vi "Sensor de Flujo_HEGO_2.vi"() -> ()   [LabVIEW 2015]
uses:
  <vilib>/MakerHub/LINX/Public/Peripherals/Digital/Digital Read N Chans.vi
  <vilib>/MakerHub/LINX/Private/Local IO/LinxDigitalRead.vi
  <vilib>/MakerHub/LINX/Public/Utilities/Check Channel.vi
  <vilib>/MakerHub/LINX/Public/Utilities/Open Serial.vi
  <vilib>/MakerHub/LINX/Private/Utilties/Generate Error.vi
  <vilib>/ptbypt/NI_PtbyPt.lvlib
  <vilib>/MakerHub/LINX/LMH-LINX.lvlib
panel:
  out "x+y":dbl
  in  "Guardar datos a excel":bool
  out "Flujo de Salida":dbl
  in  "Rango de Grafica (tiempo)":u32(knob) scale=0.0..100.0
  in  "tiempo de muestreo":dbl(knob)=0.2 caption="Time Target (s)" scale=0.0..1.0
  out "Numeric 2":i32
  out "NumdePulsos2":i32
  out "XY Graph":cluster{dbl[], dbl[]}[](graph) caption="Flujo de Entrada y Salida"
  out "Loop Rate (Hz)":u32
  in  "Pin del Sensor 2":u8
  in  "Pin del Sensor 1":u8
  in  "Puerto Serial":refnum<visa-resource-name>
  in  "?":bool
  out "Flujo de Entrada":dbl
  out "Numero de puls":i32
  out "NumdePulsos1":i32
  # "MONITOREO DE FLUJO ATRAVEZ DEL SENSOR YF-S201"
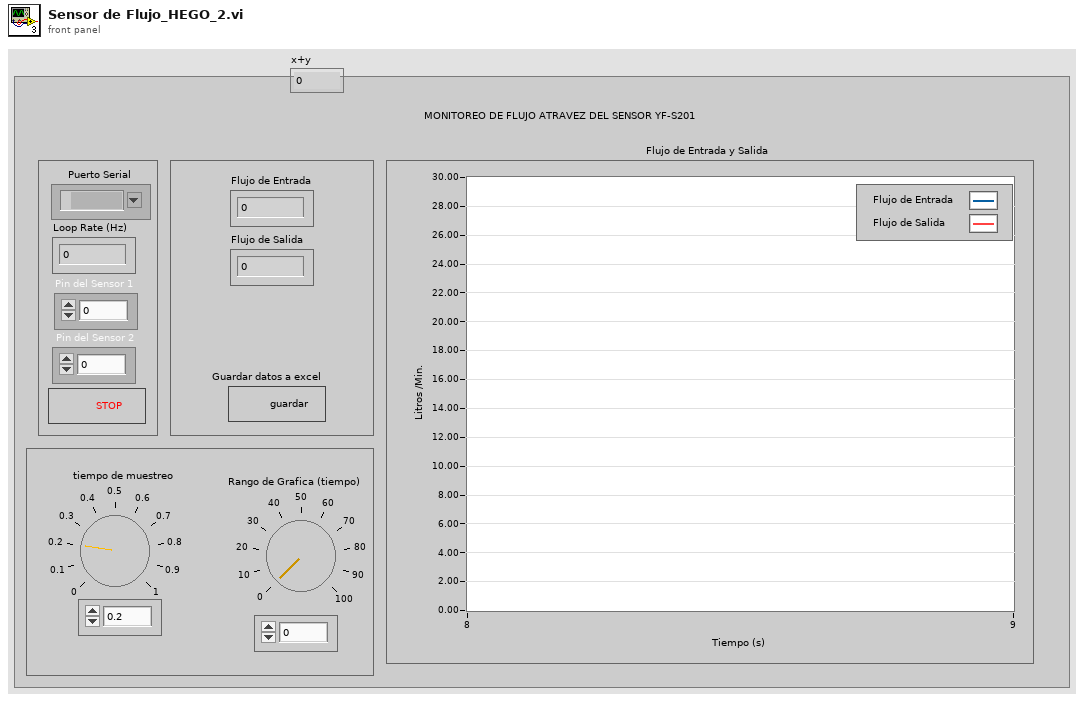
[diagram p1: front panel]
types:
  T1 = typedef "LMH-LINX.lvlib/LINX Ref.ctl" = cluster{"IO":T2, "Interface":T3, "LINX Device Config":T4}
  T2 = typedef "LMH-LINX.lvlib/Platform.ctl" = enum16{"Remote", "Local"}
  T3 = typedef "LMH-LINX.lvlib/Interface.ctl" = enum16{"Serial", "TCP"}
  T4 = typedef "LMH-LINX.lvlib/Device.lvlib/LINX Device Config.ctl" = cluster{"Interface":T3, "COM Port":refnum<visa-resource-name>, "TCP Configuration":T5, "Device Family":u8, "Device ID":u8, "Device Name":string, "TCP Ref":refnum<k5>, "Channels":T6}
  T5 = typedef "LMH-LINX.lvlib/Device.lvlib/TCP Config.ctl" = cluster{"IP Address":string, "Port":u16}
  T6 = typedef "LMH-LINX.lvlib/Channels.ctl" = cluster{"DI":u8[], "DO":u8[], "AI":u8[], "AO":u8[], "PWM":u8[], "QE":u8[], "UART":u8[], "I2C 2":u8[], "SPI":u8[], "CAN":u8[], "Servo":u8[], "AI Ref (V)":dbl, "AI Resolution (Bits)":u8, "AO Ref (V)":dbl, "AO Resolution (Bits)":u8}
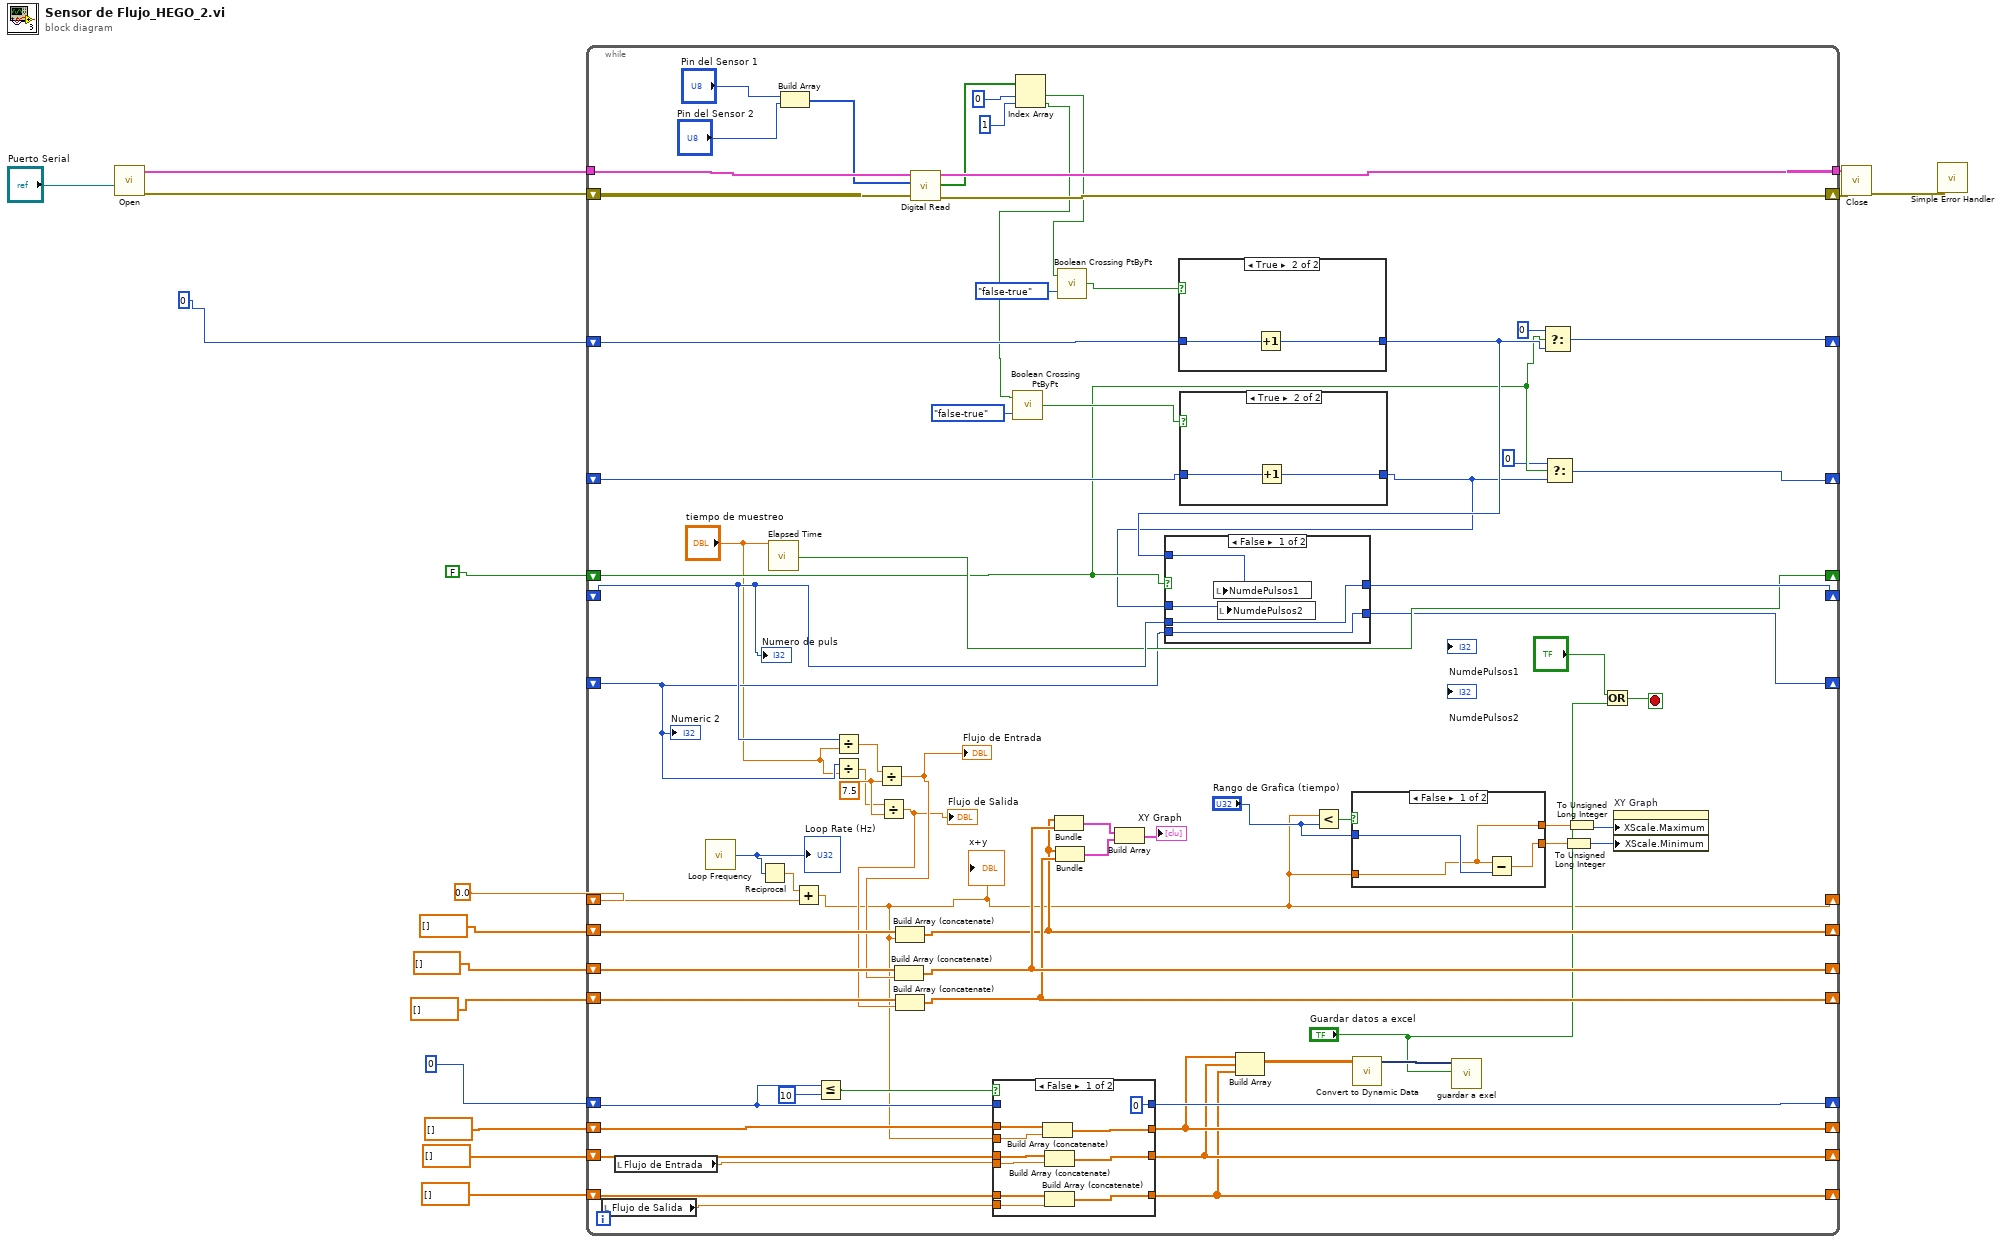
[diagram p0: block diagram]
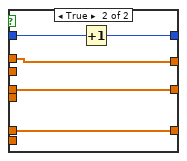
[diagram p2: hidden frame]
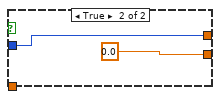
[diagram p3: hidden frame]
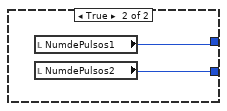
[diagram p5: hidden frame]
diagram:
  n1 = call-poly <vilib>:"Open.vi"("Serial Port"="Puerto Serial") -> ("Error Out"=w15:errorcluster, "LINX Resource"=w16:T1)  [unwired: 8 in, 1 out]
  n2 = while {
    tunnel: w16 -> [w80]
    tunnel: [w81] -> w13
    shift-right: [w83] -> _
    shift-left: 0 ("CONTADOR 2") -> [w86]
    shift-right: [w82] -> _
    shift-left: _ -> [w69]
    shift-right: [w57] -> _
    shift-left: _ -> [w70]
    shift-right: [w68] -> _
    shift-left: FALSE -> [w59]
    shift-right: [w17] -> _
    shift-left: 0.0 -> [w65]
    shift-right: [w43] -> _
    shift-left: dbl[] [] -> [w64]
    shift-right: [w61] -> _
    shift-left: dbl[] [] -> [w63]
    shift-right: [w60] -> _
    shift-left: _ -> [w54]
    shift-right: [w49] -> _
    shift-left: dbl[] [] ("Numeric") -> [w51]
    shift-right: [w44] -> w5
    shift-left: w15 -> [w79]
    shift-right: [w31] -> _
    shift-left: dbl[] [] ("Numeric") -> [w36]
    shift-right: [w32] -> _
    shift-left: dbl[] [] -> [w38]
    shift-right: [w33] -> _
    shift-left: dbl[] [] -> [w37]
    shift-right: [w34] -> _
    shift-left: 0 -> [w35]
    stop <- w28 stop-if-true
    w53 = 7.5
    n3 = local read "Flujo de Salida"() -> (w29:dbl)
    n4 = local read "Flujo de Entrada"() -> (w30:dbl)
    n5 = call <vilib>:"Loop Frequency.vi"() -> ("Loop Rate (Hz)"=w67:u32)
    "Loop Rate (Hz)" <- w67
    n6 = Reciprocal(x=w67) -> (1/x=w66:dbl)
    n7 = call "Elapsed Time"("Time Target (s)"="tiempo de muestreo") -> ("Time has Elapsed"=w68:bool)  [unwired: 11 in, 7 out]
    n8 = Build Array("Pin del Sensor 1", "Pin del Sensor 2") -> (w75:u8[])
    n9 = Add(x=w66, y=w65) -> (x+y=w17:dbl)
    "x+y" <- w17
    n10 = Less Or Equal?(x=w35, y=u32 10) -> (x <= y?=w23:bool)
    n11 = Divide(x=w69, y="tiempo de muestreo") -> (x/y=w55:dbl)
    n12 = Divide(x=w54, y="tiempo de muestreo") -> (x/y=w52:dbl)
    n13 = Divide(x=w55, y=w53) -> (x/y=w62:dbl)
    "Flujo de Entrada" <- w62
    n14 = Divide(x=w52, y=w53) -> (x/y=w42:dbl)
    "Flujo de Salida" <- w42
    n15 = Build Array (concatenate)(w63, w62) -> (w61:dbl[])
    n16 = Build Array (concatenate)(w64, w17) -> (w43:dbl[])
    n17 = Build Array (concatenate)(w51, w42) -> (w49:dbl[])
    n18 = call-poly <vilib>:"Digital Read.vi"("Error In"=w79, "DI Channels"=w75, "LINX Resource"=w80) -> ("Error Out"=w44:errorcluster, "Values"=w74:bool[], "LINX Resource"=w81:T1)  [unwired: 6 in]
    n19 = case shown="False" w23 {
      tunnel: w35 -> [_ w103]
      tunnel: [u32 0 w102] -> w34
      tunnel: w37 -> [w97 w99]
      tunnel: w30 -> [w95 _]
      tunnel: [w98 w101] -> w32
      tunnel: w38 -> [w96 w101]
      tunnel: w29 -> [w93 _]
      tunnel: w36 -> [w94 w100]
      tunnel: [w92 w100] -> w31
      tunnel: [w91 w99] -> w33
      tunnel: w17 -> [w90 _]
      frame False {
        n20 = Build Array (concatenate)(w97, w90) -> (w91:dbl[])
        n21 = Build Array (concatenate)(w96, w95) -> (w98:dbl[])
        n22 = Build Array (concatenate)(w94, w93) -> (w92:dbl[])
      }
      frame True {
        n23 = Increment(x=w103) -> (x+1=w102:u32)
      }
    }
    n24 = Index Array(array=w74, index #1=0 ("index"), index #2=1 ("index")) -> (element #1=w25:bool, element #2=w24:bool)
    n25 = call <vilib>:"Boolean Crossing PtByPt.vi"("direction"=enum16{"either", "false-true", "true-false"}."false-true", "input"=w24) -> ("crossing"=w71:bool)  [unwired: 1 in]
    n26 = Bundle(w43, w61) -> (w50:cluster{dbl[], dbl[]})  [unwired: 1 in]
    n27 = Bundle(w43, w49) -> (w48:cluster{dbl[], dbl[]})  [unwired: 1 in]
    n28 = call <vilib>:"Boolean Crossing PtByPt.vi"("direction"=enum16{"either", "false-true", "true-false"}."false-true", "input"=w25) -> ("crossing"=w87:bool)  [unwired: 1 in]
    n29 = Build Array(w50, w48) -> (→"XY Graph":cluster{dbl[], dbl[]}[])
    n30 = case shown="True" w87 {
      tunnel: w86 -> [w118 w120]
      tunnel: [w118 w119] -> w84
      frame False {
      }
      frame True {
        n31 = Increment(x=w120) -> (x+1=w119:i32)
      }
    }
    n32 = case shown="True" w71 {
      tunnel: w70 -> [w109 w111]
      tunnel: [w109 w110] -> w56
      frame False {
      }
      frame True {
        n33 = Increment(x=w111) -> (x+1=w110:i32)
      }
    }
    n34 = case shown="False" w59 {
      tunnel: w84 -> [w115 _]
      tunnel: [w114 w117] -> w82
      tunnel: w69 -> [w114 _]
      tunnel: w56 -> [w113 _]
      tunnel: [w112 w116] -> w60
      tunnel: w54 -> [w112 _]
      frame False {
        n35 = local write "NumdePulsos1"(w115) -> ()
        n36 = local write "NumdePulsos2"(w113) -> ()
      }
      frame True {
        n37 = local read "NumdePulsos1"() -> (w117:i32)
        n38 = local read "NumdePulsos2"() -> (w116:i32)
      }
    }
    n39 = Build Array(w33, w32, w31) -> (w39:dbl[][])
    n40 = Less?(x=w17, y="Rango de Grafica (tiempo)") -> (x < y?=w45:bool)
    n41 = case shown="False" w45 {
      tunnel: [w104 w107] -> w21
      tunnel: [w106 0.0] -> w20
      tunnel: w17 -> [w104 _]
      tunnel: "Rango de Grafica (tiempo)" -> [w105 w107]
      frame False {
        n42 = Subtract(x=w104, y=w105) -> (x-y=w106:dbl)
      }
      frame True {
      }
    }
    n43 = call "Convert to Dynamic Data"("2D Array"=w39) -> ("Dynamic Data Type"=w40:dynamicdata)  [unwired: 3 in]
    n44 = call "guardar a exel"("Signals"=w40, "Enable"="Guardar datos a excel") -> ()  [unwired: 15 in, 3 out]
    n45 = Select(t=0, s=w59, f=w84) -> (s? t:f=w83:i32)
    n46 = Select(t=0, s=w59, f=w56) -> (s? t:f=w57:i32)
    n47 = To Unsigned Long Integer(number=w20) -> (unsigned 32bit integer=w19:u32)
    n48 = To Unsigned Long Integer(number=w21) -> (unsigned 32bit integer=w18:u32)
    n49 = Or(x="?", y="Guardar datos a excel") -> (x .or. y?=w28:bool)
    n50 = property on="XY Graph" class="XYGraph (strict)"("XScale.Maximum"=w18, "XScale.Minimum"=w19) -> ()  [unwired: 2 in, 2 out]
    "Numero de puls" <- w69
    "Numeric 2" <- w54
  }
  n51 = call <vilib>:"Close.vi"("Error In"=w5, "LINX Resource"=w13) -> ("Error Out"=w12:errorcluster)  [unwired: 9 in]
  n52 = call <vilib>:"Simple Error Handler.vi"("error in (no error)"=w12) -> ()  [unwired: 4 in, 5 out]
